vi "Run.vi"(8 "error in (no error)":errorcluster, 11 "Channel GUI in":refnum<class "Channel GUI.lvclass">) -> (0 "error out":errorcluster, 3 "Channel GUI out":refnum<class "Channel GUI.lvclass">)   [LabVIEW 2018, in "Channel GUI.lvclass"]
uses:
  Channel GUI.lvclass
  Channel GUI.lvclass/Channel GUI.ctl
  State Machine/State Machine.lvclass
  Stream/Stream.lvclass
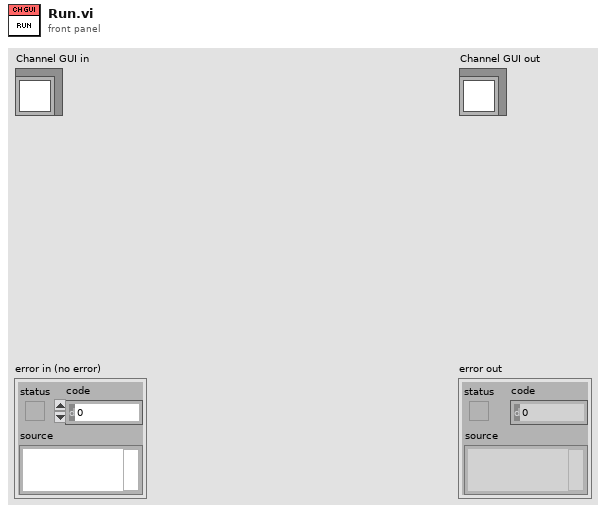
[diagram p1: front panel]
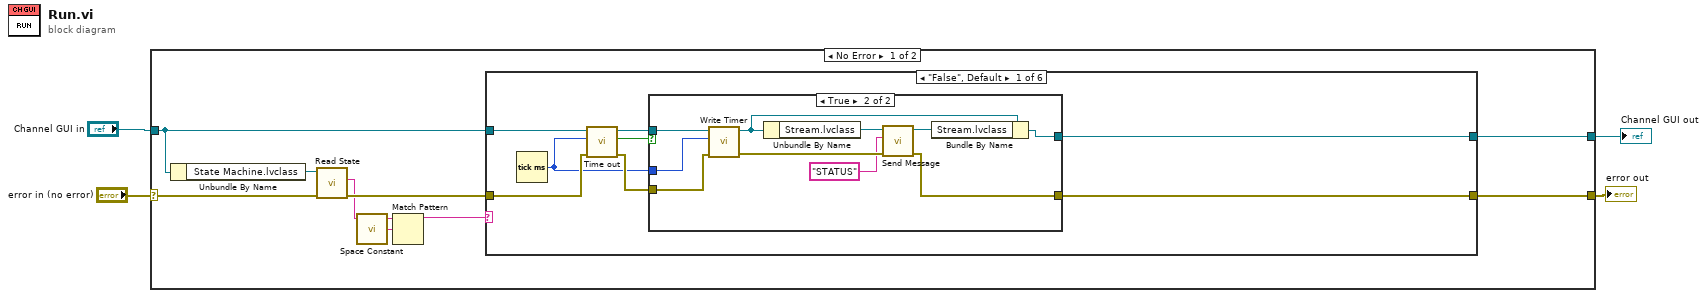
[diagram p0: block diagram]
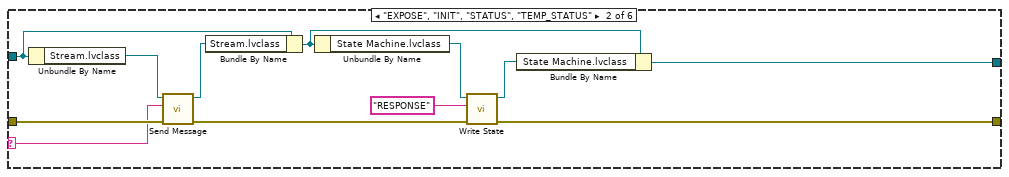
[diagram p3: hidden frame]
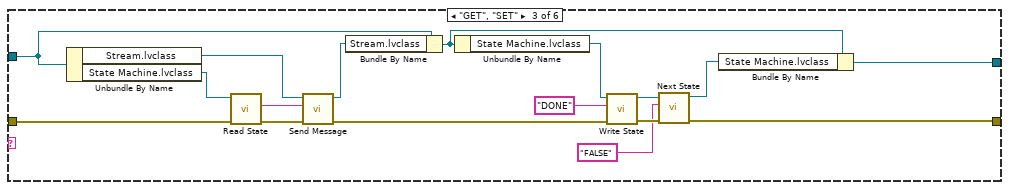
[diagram p4: hidden frame]
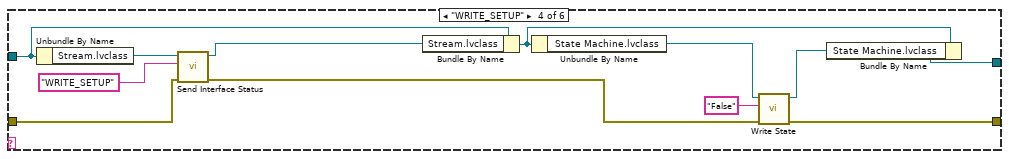
[diagram p5: hidden frame]
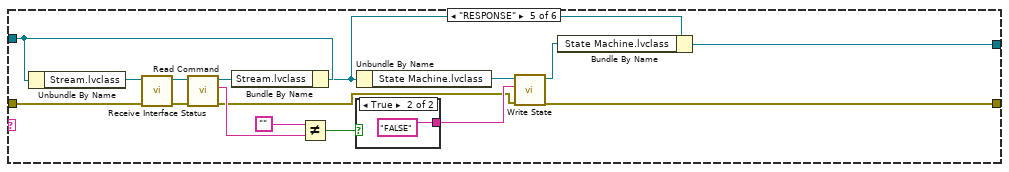
[diagram p6: hidden frame]
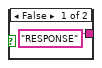
[diagram p7: hidden frame]
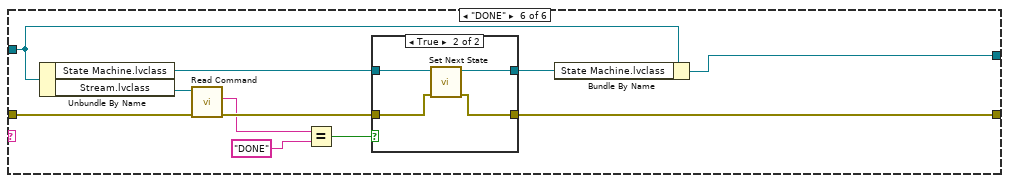
[diagram p8: hidden frame]
diagram:
  n1 = case shown="No Error" "error in (no error)" {
    selector: "error in (no error)" -> [w11 w111]
    tunnel: [w13 w111] -> w2
    tunnel: "Channel GUI in" -> [w9 w110]
    tunnel: [w5 w110] -> w1
    frame No Error {
      n2 = Unbundle By Name(w9) -> ("State Machine.lvclass"=w12:refnum<class "State Machine.lvclass">)
      n3 = call-dynamic "Read State.vi"("error in (no error)"=w11, "State Machine in"=w12) -> ("error out"=w10:errorcluster, "State"=w7:string)  [unwired: 7 in, 1 out]
      n4 = call <vilib>:"Space Constant.vi"() -> ("String"=w8:string)
      n5 = Match Pattern(string=w7, regular expression=w8) -> (before substring=w6:string)  [unwired: 1 in, 3 out]
      n6 = case shown="\"False\", Default" w6 {
        selector: w6 -> [_ w34 _ _ _ _]
        tunnel: w10 -> [w21 w44 w47 w66 w83 w102]
        tunnel: [w17 w37 w51 w70 w89 w94] -> w13
        tunnel: w9 -> [w15 w43 w56 w72 w90 w96]
        tunnel: [w16 w40 w57 w71 w86 w93] -> w5
        frame "False", Default {
          n7 = Tick Count (ms)() -> (millisecond timer value=w18:u32)
          n8 = call "Time out.vi"("error in (no error)"=w21, "New Time"=w18, "Channel GUI in"=w15) -> ("error out"=w19:errorcluster, "time out ?"=w14:bool, "Channel GUI out"=w20:refnum<class "Channel GUI.lvclass">)  [unwired: 6 in]
          n9 = case shown="True" w14 {
            tunnel: w20 -> [w23 w26]
            tunnel: w19 -> [w22 w33]
            tunnel: w18 -> [_ w32]
            tunnel: [w22 w28] -> w17
            tunnel: [w23 w27] -> w16
            frame False {
            }
            frame True {
              n10 = call "Write Timer.vi"("error in (no error)"=w33, "Timer"=w32, "Channel GUI in"=w26) -> ("error out"=w30:errorcluster, "Channel GUI out"=w24:refnum<class "Channel GUI.lvclass">)  [unwired: 7 in]
              n11 = Unbundle By Name(w24) -> ("Stream.lvclass"=w25:refnum<class "Stream.lvclass">)
              n12 = call "Send Message.vi"("error in (no error)"=w30, "Message"="STATUS" ("New_State"), "Stream in"=w25) -> ("error out"=w28:errorcluster, "Stream out"=w31:refnum<class "Stream.lvclass">)  [unwired: 7 in]
              n13 = Bundle By Name(cluster=w24, "Stream.lvclass"=w31) -> (w27:refnum<class "Channel GUI.lvclass">)
            }
          }
        }
        frame "EXPOSE", "INIT", "STATUS", "TEMP_STATUS" {
          n14 = Unbundle By Name(w43) -> ("Stream.lvclass"=w45:refnum<class "Stream.lvclass">)
          n15 = call "Send Message.vi"("error in (no error)"=w44, "Message"=w34, "Stream in"=w45) -> ("error out"=w36:errorcluster, "Stream out"=w42:refnum<class "Stream.lvclass">)  [unwired: 7 in]
          n16 = Bundle By Name(cluster=w43, "Stream.lvclass"=w42) -> (w41:refnum<class "Channel GUI.lvclass">)
          n17 = Unbundle By Name(w41) -> ("State Machine.lvclass"=w39:refnum<class "State Machine.lvclass">)
          n18 = call-dynamic "Write State.vi"("error in (no error)"=w36, "State"="RESPONSE" ("New_State"), "State Machine in"=w39) -> ("error out"=w37:errorcluster, "State Machine out"=w38:refnum<class "State Machine.lvclass">)  [unwired: 7 in]
          n19 = Bundle By Name(cluster=w41, "State Machine.lvclass"=w38) -> (w40:refnum<class "Channel GUI.lvclass">)
        }
        frame "GET", "SET" {
          n20 = Unbundle By Name(w56) -> ("Stream.lvclass"=w59:refnum<class "Stream.lvclass">, "State Machine.lvclass"=w49:refnum<class "State Machine.lvclass">)
          n21 = call-dynamic "Read State.vi"("error in (no error)"=w47, "State Machine in"=w49) -> ("error out"=w48:errorcluster, "State"=w46:string)  [unwired: 7 in, 1 out]
          n22 = call "Send Message.vi"("error in (no error)"=w48, "Message"=w46, "Stream in"=w59) -> ("error out"=w62:errorcluster, "Stream out"=w60:refnum<class "Stream.lvclass">)  [unwired: 7 in]
          n23 = Bundle By Name(cluster=w56, "Stream.lvclass"=w60) -> (w61:refnum<class "Channel GUI.lvclass">)
          n24 = Unbundle By Name(w61) -> ("State Machine.lvclass"=w55:refnum<class "State Machine.lvclass">)
          n25 = call-dynamic "Write State.vi"("error in (no error)"=w62, "State"="DONE" ("New_State"), "State Machine in"=w55) -> ("error out"=w54:errorcluster, "State Machine out"=w53:refnum<class "State Machine.lvclass">)  [unwired: 7 in]
          n26 = call "Next State.vi"("error in (no error)"=w54, "New_State"="FALSE", "State Machine in"=w53) -> ("error out"=w51:errorcluster, "State Machine out"=w52:refnum<class "State Machine.lvclass">)  [unwired: 7 in]
          n27 = Bundle By Name(cluster=w61, "State Machine.lvclass"=w52) -> (w57:refnum<class "Channel GUI.lvclass">)
        }
        frame "WRITE_SETUP" {
          n28 = Unbundle By Name(w72) -> ("Stream.lvclass"=w67:refnum<class "Stream.lvclass">)
          n29 = call "Send Interface Status.vi"("error in (no error)"=w66, "Message"="WRITE_SETUP" ("New_State"), "Stream in"=w67) -> ("error out"=w63:errorcluster, "Stream out"=w64:refnum<class "Stream.lvclass">)  [unwired: 7 in]
          n30 = Bundle By Name(cluster=w72, "Stream.lvclass"=w64) -> (w73:refnum<class "Channel GUI.lvclass">)
          n31 = Unbundle By Name(w73) -> ("State Machine.lvclass"=w74:refnum<class "State Machine.lvclass">)
          n32 = call-dynamic "Write State.vi"("error in (no error)"=w63, "State"="False" ("New_State"), "State Machine in"=w74) -> ("error out"=w70:errorcluster, "State Machine out"=w69:refnum<class "State Machine.lvclass">)  [unwired: 7 in]
          n33 = Bundle By Name(cluster=w73, "State Machine.lvclass"=w69) -> (w71:refnum<class "Channel GUI.lvclass">)
        }
        frame "RESPONSE" {
          n34 = Unbundle By Name(w90) -> ("Stream.lvclass"=w84:refnum<class "Stream.lvclass">)
          n35 = call "Receive Interface Status.vi"("error in (no error)"=w83, "Stream in"=w84) -> ("error out"=w82:errorcluster, "Stream out"=w81:refnum<class "Stream.lvclass">)  [unwired: 8 in]
          n36 = call "Read Command.vi"("error in (no error)"=w82, "Stream in"=w81) -> ("error out"=w75:errorcluster, "Command"=w80:string, "Stream out"=w77:refnum<class "Stream.lvclass">)  [unwired: 7 in]
          n37 = Bundle By Name(cluster=w90, "Stream.lvclass"=w77) -> (w87:refnum<class "Channel GUI.lvclass">)
          n38 = Not Equal?(x="", y=w80) -> (x != y?=w78:bool)
          n39 = case shown="True" w78 {
            tunnel: ["RESPONSE" "FALSE"] -> w76
            frame False {
            }
            frame True {
            }
          }
          n40 = Unbundle By Name(w87) -> ("State Machine.lvclass"=w88:refnum<class "State Machine.lvclass">)
          n41 = call-dynamic "Write State.vi"("error in (no error)"=w75, "State"=w76, "State Machine in"=w88) -> ("error out"=w89:errorcluster, "State Machine out"=w85:refnum<class "State Machine.lvclass">)  [unwired: 7 in]
          n42 = Bundle By Name(cluster=w87, "State Machine.lvclass"=w85) -> (w86:refnum<class "Channel GUI.lvclass">)
        }
        frame "DONE" {
          n43 = Unbundle By Name(w96) -> ("State Machine.lvclass"=w97:refnum<class "State Machine.lvclass">, "Stream.lvclass"=w103:refnum<class "Stream.lvclass">)
          n44 = call "Read Command.vi"("error in (no error)"=w102, "Stream in"=w103) -> ("error out"=w101:errorcluster, "Command"=w98:string)  [unwired: 7 in, 1 out]
          n45 = Equal?(x=w98, y="DONE") -> (x = y?=w100:bool)
          n46 = case shown="True" w100 {
            tunnel: [w105 w106] -> w94
            tunnel: w101 -> [w105 w107]
            tunnel: w97 -> [w104 w109]
            tunnel: [w104 w108] -> w95
            frame False {
            }
            frame True {
              n47 = call "Set Next State.vi"("error in (no error)"=w107, "State Machine in"=w109) -> ("error out"=w106:errorcluster, "State Machine out"=w108:refnum<class "State Machine.lvclass">)  [unwired: 8 in]
            }
          }
          n48 = Bundle By Name(cluster=w96, "State Machine.lvclass"=w95) -> (w93:refnum<class "Channel GUI.lvclass">)
        }
      }
    }
    frame Error {
    }
  }
  "error out" <- w2
  "Channel GUI out" <- w1
